vi "HB_ConfigureDIO.vi"(6 "Value":bool, 8 "error in (no error)":errorcluster, 9 "Direction":bool, 10 "DIO Channel":T1=enum."HB GPIO 0", 11 "HBDeviceRef":T2) -> (0 "error out":errorcluster, 2 "Received":string, 3 "HBDeviceRef":T2)   [LabVIEW 2018]
doc: "Sets the specified digital channel to either input or output. If the channel is set to output, it is also set to the specified value where true corresponds to a high signal and false to low. Only a subset of channels may be configured as DIO channels; this is enforced by the DIO Channel typedef."
uses:
  <vilib>/Rock Robotics/WPI/SerialPort/WPI_SerialPortRef.ctl
  <vilib>/Rock Robotics/WPI/ThirdParty/Sensors/Huskie Board SDK for LabVIEW 2.0.0/Huskie Board SDK for LabVIEW/Huskie Board/DIO Channels.ctl
  <vilib>/Utility/error.llb/Error Cluster From Error Code.vi
  <vilib>/ErrorRing/Error Ring.xnode
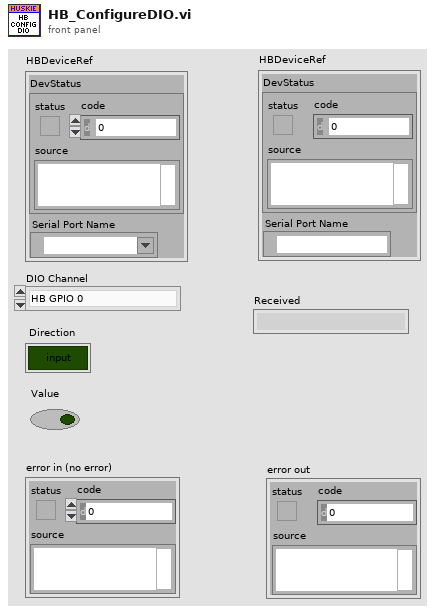
[diagram p1: front panel]
types:
  T1 = typedef "DIO Channels.ctl" = enum8{"SD card D1", "SD card D0", "SD card CLK", "SD card CMD", "SD card D2", "SD card D3", "roboRIO MOSI", "roboRIO MISO", "roboRIO CLK", "roboRIO CS", "roboRIO UART RX", "roboRIO UART TX", "roboRIO SCL", "robotRIO SDA", "HB GPIO 0", "HB GPIO 1", "HB GPIO 2", "HB GPIO 3", "HB LCD", "ADC CS2", "ADC CS1", "ADC DO", "ADC CLK", "ADC DI", "LED 1", "LED 2", "LED 3", "LED 4", "EEPROM SCL", "EEPROM SDA", "USB UART TX", "USB UART RX"}
  T2 = typedef "WPI_SerialPortRef.ctl" = cluster{"DevStatus":errorcluster, "Serial Port Name":refnum<visa-resource-name>}
  T3 = enum8{"SD card D1", "SD card D0", "SD card CLK", "SD card CMD", "SD card D2", "SD card D3", "roboRIO MOSI", "roboRIO MISO", "roboRIO CLK", "roboRIO CS", "roboRIO UART RX", "roboRIO UART TX", "roboRIO SCL", "robotRIO SDA", "HB GPIO 0", "HB GPIO 1", "HB GPIO 2", "HB GPIO 3", "HB LCD", "ADC CS2", "ADC CS1", "ADC DO", "ADC CLK", "ADC DI", "LED 1", "LED 2", "LED 3", "LED 4", "EEPROM SCL", "EEPROM SDA", "USB UART TX", "USB UART RX"}[]
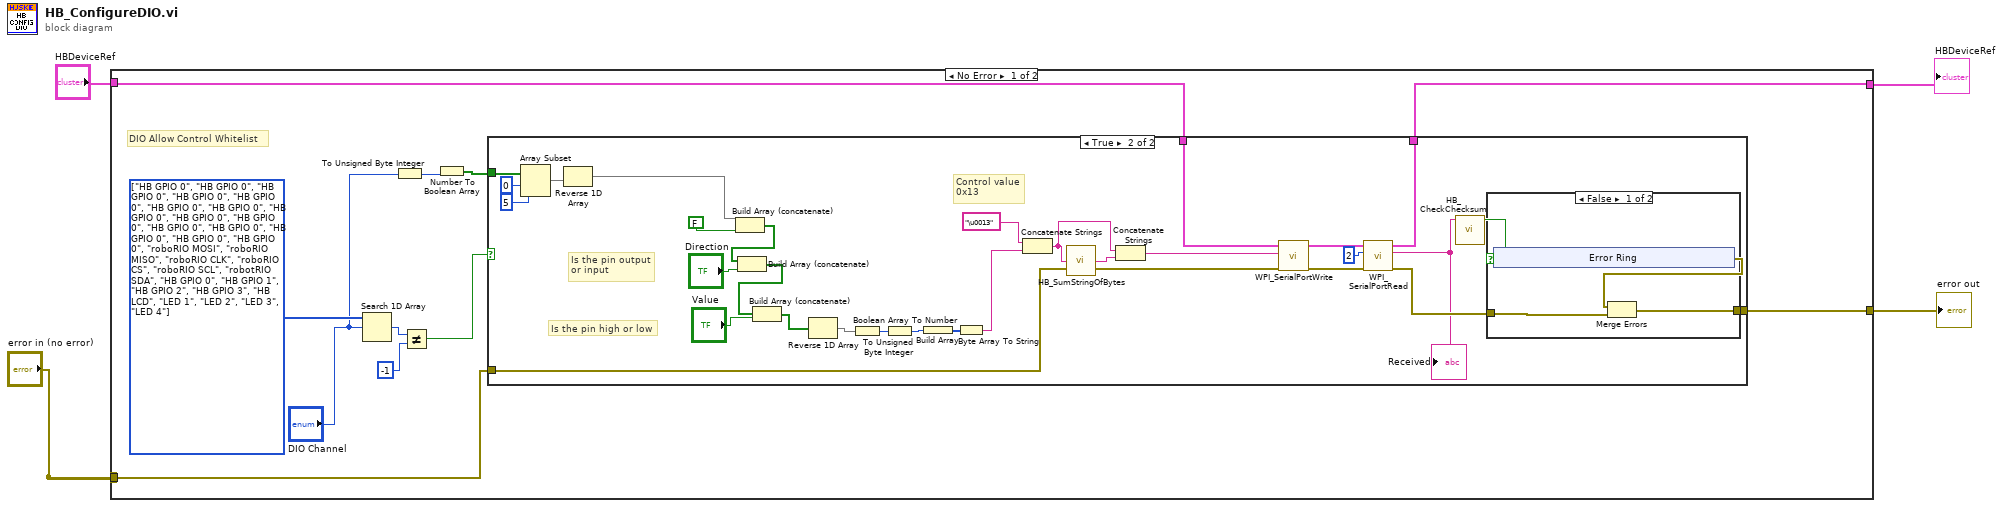
[diagram p0: block diagram]
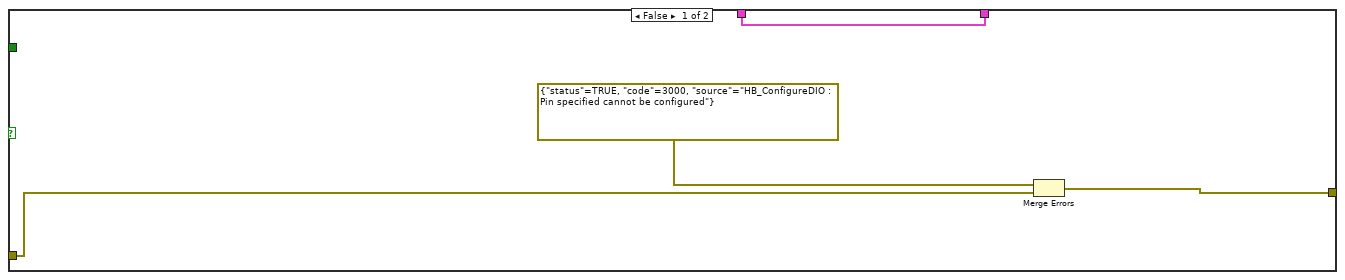
[diagram p2: hidden frame]
diagram:
  n1 = case shown="No Error" "error in (no error)" {
    selector: "error in (no error)" -> [_ w58]
    tunnel: "HBDeviceRef" -> [w15 w59]
    tunnel: "error in (no error)" -> [w14 _]
    tunnel: [w13 w59] -> w3
    tunnel: [w10 w58] -> w2
    frame No Error {
      w9 = T3 [enum."HB GPIO 0", enum."HB GPIO 0", enum."HB GPIO 0", enum."HB GPIO 0", enum."HB GPIO 0", enum."HB GPIO 0", enum."HB GPIO 0", enum."HB GPIO 0", enum."HB GPIO 0", enum."HB GPIO 0", enum."HB GPIO 0", enum."HB GPIO 0", enum."HB GPIO 0", enum."HB GPIO 0", enum."HB GPIO 0", enum."roboRIO MOSI", enum."roboRIO MISO", enum."roboRIO CLK", enum."roboRIO CS", enum."roboRIO SCL", enum."robotRIO SDA", enum."HB GPIO 0", enum."HB GPIO 1", enum."HB GPIO 2", enum."HB GPIO 3", enum."HB LCD", enum."LED 1", enum."LED 2", enum."LED 3", enum."LED 4"] items=["SD card D1", "SD card D0", "SD card CLK", "SD card CMD", "SD card D2", "SD card D3", "roboRIO MOSI", "roboRIO MISO", "roboRIO CLK", "roboRIO CS", "roboRIO UART RX", "roboRIO UART TX", "roboRIO SCL", "robotRIO SDA", "HB GPIO 0", "HB GPIO 1", "HB GPIO 2", "HB GPIO 3", "HB LCD", "ADC CS2", "ADC CS1", "ADC DO", "ADC CLK", "ADC DI", "LED 1", "LED 2", "LED 3", "LED 4", "EEPROM SCL", "EEPROM SDA", "USB UART TX", "USB UART RX"]
      # "DIO Allow Control Whitelist"
      n2 = Search 1D Array(1D array=w9, element="DIO Channel") -> (index of element=w8:i32)  [unwired: 1 in]
      n3 = To Unsigned Byte Integer(number="DIO Channel") -> (unsigned 8bit integer=w12:u8)
      n4 = Not Equal?(x=w8, y=-1) -> (x != y?=w6:bool)
      n5 = Number To Boolean Array(number=w12) -> (Boolean array=w11:bool[])
      n6 = case shown="True" w6 {
        tunnel: w15 -> [w19 w49]
        tunnel: w14 -> [w17 w48]
        tunnel: [w19 w45] -> w13
        tunnel: w11 -> [_ w37]
        tunnel: [w16 w24] -> w10
        frame False {
          n7 = Merge Errors(errorcluster {"status"=TRUE, "code"=3000, "source"="HB_ConfigureDIO : Pin specified cannot be configured"} ("error in"), w17) -> (w16:errorcluster)
        }
        frame True {
          # "Is the pin high or low"
          # "Is the pin output\nor input"
          # "Control value\n0x13"
          n8 = Array Subset(array=w37, index=0, length=5) -> (w38:bool[])
          n9 = Reverse 1D Array(array=w38) -> (reversed array=w36:bool[])
          n10 = Build Array (concatenate)(w36, FALSE ("new element/subarray")) -> (w34:bool[])
          n11 = Build Array (concatenate)(w34, "Direction") -> (w31:bool[])
          n12 = Build Array (concatenate)(w31, "Value") -> (w30:bool[])
          n13 = Reverse 1D Array(array=w30) -> (reversed array=w29:bool[])
          n14 = Boolean Array To Number(Boolean array=w29) -> (number=w43:u32)
          n15 = To Unsigned Byte Integer(number=w43) -> (unsigned 8bit integer=w42:u8)
          n16 = Build Array(w42) -> (w41:u8[])
          n17 = Byte Array To String(unsigned byte array=w41) -> (string=w27:string)
          n18 = Concatenate Strings("\u0013" ("Buffer"), w27) -> (w20:string)
          n19 = call <vilib>:"HB_SumStringOfBytes.vi"("String Of Bytes"=w20) -> ("Sum as String"=w21:string)
          n20 = Concatenate Strings(w20, w21) -> (w26:string)
          n21 = call <vilib>:"WPI_SerialPortWrite.vi"("error in (no error)"=w48, "Buffer"=w26, "SerialPortRef"=w49) -> ("error out"=w46:errorcluster, "SerialPortRef"=w47:T2)  [unwired: 6 in, 1 out]
          n22 = call <vilib>:"WPI_SerialPortRead.vi"("error in (no error)"=w46, "Num Bytes to Read"=u32 2, "SerialPortRef"=w47) -> ("error out"=w25:errorcluster, "Buffer"=w23:string, "SerialPortRef"=w45:T2)  [unwired: 6 in]
          "Received" <- w23
          n23 = call <vilib>:"HB_CheckChecksum.vi"("String"=w23) -> ("Checksum Matches"=w22:bool)  [unwired: 9 in, 1 out]
          n24 = case shown="False" w22 {
            tunnel: w25 -> [w52 w57]
            tunnel: [w51 w57] -> w24
            frame False {
              n25 = xnode "Error Ring"() -> ("error out"=w50:errorcluster)
              n26 = Merge Errors(w50, w52) -> (w51:errorcluster)
            }
            frame True {
            }
          }
        }
      }
    }
    frame Error {
    }
  }
  "HBDeviceRef" <- w3
  "error out" <- w2
